vi "InTake Finish.vi"   [LabVIEW 2013]
types:
  T1 = typedef "WPI_MotorControlDeviceRef.ctl" = cluster{"DeviceStatus":errorcluster, "Type":enum16{"PWM", "CAN"}, "PWM":cluster{"Digital Module":T2, "PWM Channel":T3, "DeadBand":T4}, "CAN":cluster{"Device Number":u8, "Control Mode":T5, "Semaphore":T6, "Max Vout":dbl}, "Invert":bool, "TransformRef":T7, "InvTransformRef":T7}
  T2 = typedef "FPGA_TypedefDigitalModule.ctl" = enum16{"Digital Module 1", "Digital Module 2"}
  T3 = typedef "FPGA_DIOPWMChannel.ctl" = enum8{"PWM 1", "PWM 2", "PWM 3", "PWM 4", "PWM 5", "PWM 6", "PWM 7", "PWM 8", "PWM 9", "PWM 10", "Invalid"}
  T4 = typedef "WPI_PWMDeadband.ctl" = cluster{"Name":string, "maxPositivePwm":i32, "minPositivePwm":i32, "centerPwm":i32, "maxNegativePwm":i32, "minNegativePwm":i32, "angularRange":u16}
  T5 = typedef "WPI_CANJaguar_ControlMode.ctl" = enum8{"Percent VBus", "Current", "Speed", "Position", "Voltage"}
  T6 = typedef "Semaphore RefNum" = refnum<k1>
  T7 = typedef "WPI_PWMTransform_ConPane.ctl" = refnum<vi>
  T8 = typedef "WPI_DigitalInputDevRef.ctl" = cluster{"DevStatus":errorcluster, "DIO Channel":T9, "Digital Module":T2}
  T9 = typedef "FPGA_DIOChannel.ctl" = enum8{"DIO 1", "DIO 2", "DIO 3", "DIO 4", "DIO 5", "DIO 6", "DIO 7", "DIO 8", "DIO 9", "DIO 10", "DIO 11", "DIO 12", "DIO 13", "DIO 14", "Invalid"}
  T10 = typedef "WPI_GyroDevRef.ctl" = cluster{"DevStatus":errorcluster, "Analog Module":T11, "Analog Channel":T12, "Offset":dbl, "Gain (VoltsPerDegree/Second)":dbl}
  T11 = typedef "FPGA_TypedefAnalogModule.ctl" = enum16{"Analog Module 1", "Analog Module 2"}
  T12 = typedef "FPGA_AIChannel.ctl" = enum8{"AI 1", "AI 2", "AI 3", "AI 4", "AI 5", "AI 6", "AI 7", "AI 8", "Invalid"}
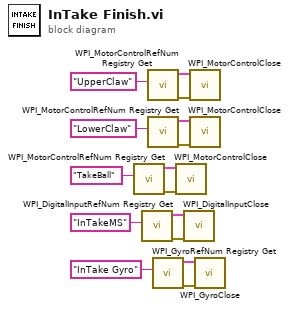
[diagram p0: block diagram]
diagram:
  n1 = call <vilib>:"WPI_MotorControlRefNum Registry Get.vi"("refnum name"="TakeBall") -> ("error out"=w11:errorcluster, "MotorControlDevRef"=w10:T1)  [unwired: 9 in]
  n2 = call <vilib>:"WPI_DigitalInputRefNum Registry Get.vi"("refnum name"="InTakeMS") -> ("error out"=w9:errorcluster, "DigitalInputDevRef"=w8:T8)  [unwired: 9 in]
  n3 = call <vilib>:"WPI_MotorControlRefNum Registry Get.vi"("refnum name"="UpperClaw") -> ("error out"=w15:errorcluster, "MotorControlDevRef"=w14:T1)  [unwired: 9 in]
  n4 = call <vilib>:"WPI_MotorControlRefNum Registry Get.vi"("refnum name"="LowerClaw") -> ("error out"=w13:errorcluster, "MotorControlDevRef"=w12:T1)  [unwired: 9 in]
  n5 = call <vilib>:"WPI_GyroRefNum Registry Get.vi"("refnum name"="InTake Gyro") -> ("error out"=w2:errorcluster, "GyroDevRef"=w1:T10)  [unwired: 9 in]
  n6 = call <vilib>:"WPI_MotorControlClose.vi"("error in (no error)"=w11, "MotorControlDevRef"=w10) -> ()  [unwired: 9 in, 1 out]
  n7 = call <vilib>:"WPI_DigitalInputClose.vi"("error in (no error)"=w9, "DigitalInputDevRef"=w8) -> ()  [unwired: 9 in, 1 out]
  n8 = call <vilib>:"WPI_MotorControlClose.vi"("error in (no error)"=w15, "MotorControlDevRef"=w14) -> ()  [unwired: 9 in, 1 out]
  n9 = call <vilib>:"WPI_MotorControlClose.vi"("error in (no error)"=w13, "MotorControlDevRef"=w12) -> ()  [unwired: 9 in, 1 out]
  n10 = call "WPI_GyroClose.vi"("error in (no error)"=w2, "GyroDevRef"=w1) -> ()  [unwired: 9 in, 1 out]
